vi "Write.vi"(8 "error in (no error)":errorcluster, 10 "DATA":T1, 11 "Queue in":refnum<class "Queue.lvclass">) -> (0 "error out":errorcluster, 3 "Queue out":refnum<class "Queue.lvclass">)   [LabVIEW 2020, in "Queue.lvclass"]
uses:
  Queue.lvclass
  Queue.lvclass/Queue.ctl
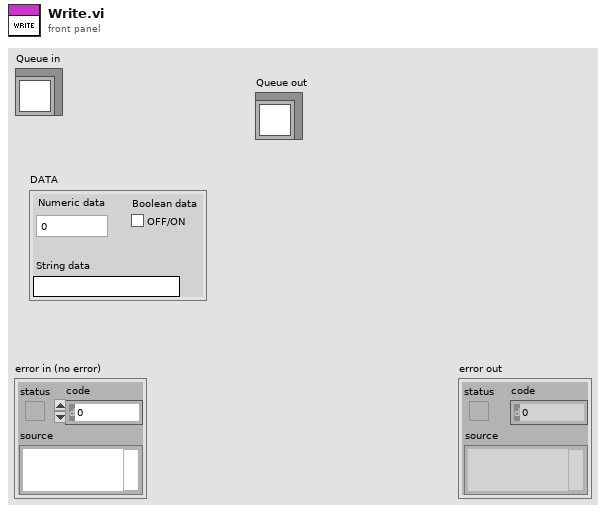
[diagram p1: front panel]
types:
  T1 = cluster{"Numeric data":dbl, "String data":string, "Boolean data":bool}
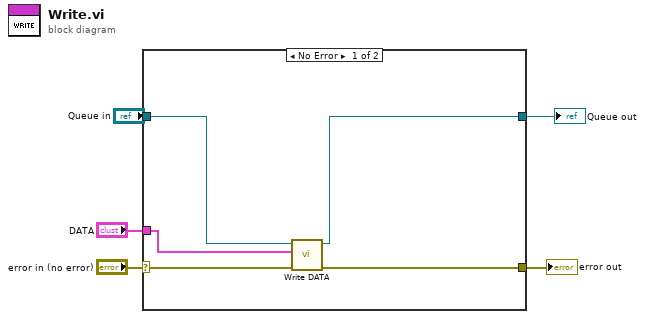
[diagram p0: block diagram]
diagram:
  n1 = case shown="No Error" "error in (no error)" {
    selector: "error in (no error)" -> [w10 w12]
    tunnel: [w9 w12] -> w4
    tunnel: [w6 w11] -> w2
    tunnel: "Queue in" -> [w8 w11]
    tunnel: "DATA" -> [w7 _]
    frame No Error {
      n2 = call "Write DATA.vi"("error in (no error)"=w10, "DATA"=w7, "Queue in"=w8) -> ("error out"=w9:errorcluster, "Queue out"=w6:refnum<class "Queue.lvclass">)  [unwired: 7 in]
    }
    frame Error {
    }
  }
  "error out" <- w4
  "Queue out" <- w2
